vi "Read Position.vi"(8 "error in":errorcluster, 11 "Switch Step in":refnum<class "Switch Step.lvclass">) -> (0 "error out":errorcluster, 2 "Position":bool, 3 "Switch Step out":refnum<class "Switch Step.lvclass">)   [LabVIEW 2018, in "Sequence Composition.lvlib" / "Switch Step.lvclass"]
uses:
  Switch Step.lvclass
  Switch Step.lvclass/Switch Step.ctl
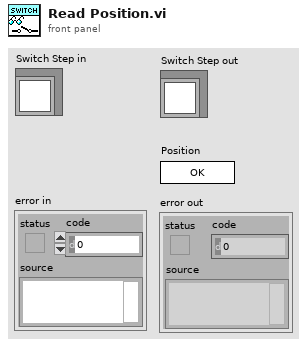
[diagram p1: front panel]
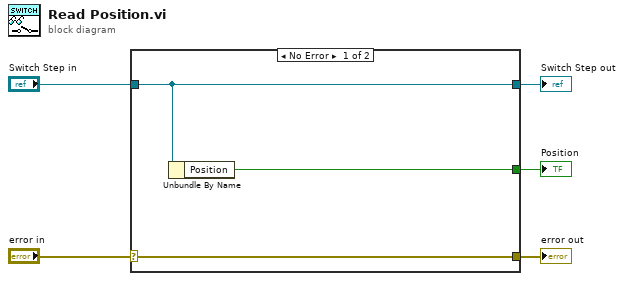
[diagram p0: block diagram]
diagram:
  n1 = case shown="No Error" "error in" {
    selector: "error in" -> [w8 w9]
    tunnel: [w8 w9] -> w4
    tunnel: [w7 w10] -> w2
    tunnel: "Switch Step in" -> [w7 w10]
    tunnel: [w6 _] -> w1
    frame No Error {
      n2 = Unbundle By Name(w7) -> ("Position"=w6:bool)
    }
    frame Error {
    }
  }
  "error out" <- w4
  "Switch Step out" <- w2
  "Position" <- w1
